vi "Create I2C Object.vi"(8 "error in (no error)":errorcluster, 11 "LCM Single-Up MTS Test in":refnum<class "LCM Single-Up MTS Test.lvclass">) -> (0 "error out":errorcluster, 3 "I2C":refnum<class "NI-8452.lvclass">)   [LabVIEW 2015, in "LCM Single-Up MTS Test.lvclass"]
uses:
  LCM Single-Up MTS Test.lvclass
  Classes/Instruments/I2C Device/NI-8452/NI-8452.lvclass
  CBTF Applications/SmartCast Testing/Main/LCM Single-Up/Application/Application/Class/typedefs/Instrument Selector -- Enum.ctl
  Classes/Application/Class/Application.lvclass
  Test Class/Test Class.lvclass
  CBTF Applications/SmartCast Testing/Main/LCM Single-Up/Application/Application/Class/LCM Single-Up.lvclass
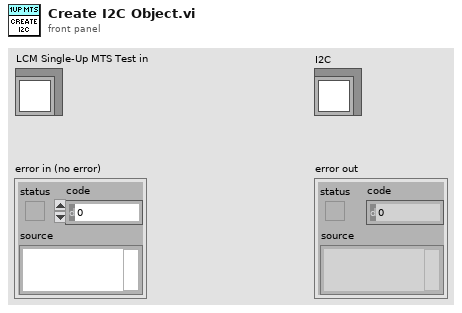
[diagram p1: front panel]
types:
  T1 = typedef "LCM Single-Up.lvlib/LCM Single-Up.lvclass/Instrument Selector -- Enum.ctl" = enum16{"Relay", "MIO Device", "I2C Device", "Thermocouple"}
  T2 = typedef "Application.lvlib/App Properties.lvclass/Class Properties -- Cluster.ctl" = cluster{"UUT Info":T3[], "Test Information":refnum<vi>, "Test Complete Event":refnum<user-event>, "Shop Floor System":refnum<class "Shop Floor System.lvclass">, "Gold Board":refnum<class "Golden Board.lvclass">, "Test Recipe":refnum<class "Test Recipe.lvclass">, "Instruments":refnum<class "Base Class.lvclass">[], "Mode":T4, "Test Results":cluster{"Pass":bool[], "Fail Codes":string[]}, "Station Config":refnum<class "Station Config.lvclass">}
  T3 = typedef "Application.lvlib/App Properties.lvclass/UUT Reference -- Cluster.ctl" = cluster{"Serial Number Reference":refnum<vi>, "Status Message Reference":refnum<vi>}
  T4 = typedef "Application.lvlib/Application.lvclass/Op Mode -- Enum.ctl" = u16
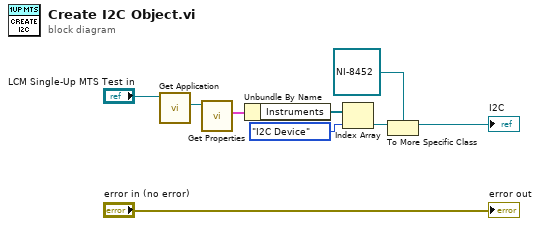
[diagram p0: block diagram]
diagram:
  n1 = call "Get Application.vi"("Test Class in"="LCM Single-Up MTS Test in") -> ("Application.lvlib:Application.lvclass"=w3:refnum<class "Application.lvclass">)  [unwired: 9 in, 1 out]
  n2 = call "Get Properties.vi"("Acrobat Template in"=w3) -> ("Class Properties"=w5:T2)  [unwired: 8 in, 2 out]
  n3 = Unbundle By Name(w5) -> ("Instruments"=w7:refnum<class "Base Class.lvclass">[])
  n4 = Index Array(array=w7, index=Instrument_Selector_--_Enum."I2C Device" ("Instrument")) -> (element=w6:refnum<class "Base Class.lvclass">)
  n5 = To More Specific Class(target class=refnum<class "NI-8452.lvclass"> refnum ("I2C"), reference=w6) -> (specific class reference=→"I2C":refnum<class "NI-8452.lvclass">)  [unwired: 1 in, 1 out]
  "error out" <- "error in (no error)"
